vi "Test New File Sink.vi"(11 "Test Case In":refnum<class "File Sink.lvclass">) -> (0 "error out":errorcluster, 3 "Test Case Out":refnum<class "File Sink.lvclass">)   [LabVIEW 2020, in "Testing.lvlib" / "File Sink.lvclass"]
uses:
  File Sink.lvclass
  C:/Program Files (x86)/National Instruments/LabVIEW 2020/vi.lib/Astemes/LUnit/Test Case.lvclass
  Source/Sinks/File Sink/File Sink.lvclass/File Sink.ctl
  <vilib>/Astemes/LUnit/Test Case.lvclass/Test Case.ctl
  4993e8ee-a06a-463a-9684-69129f64d5ce.vi
  <vilib>/Astemes/LUnit/Core/LUnit Test Case/Private/Append Pass Result.vi
  <vilib>/Astemes/LUnit/Core/LUnit Test Case/Private/Append Fail Result.vi
  4993e8ee-a06a-463a-9684-69129f64d5ce.vi/9c5d11cd-9439-4240-a1ee-d9baace9c924.vi
  <vilib>/Astemes/LUnit/Core/LUnit Test Case/Private/Run In UI.vi
  Source/Sinks/File Sink/File Sink.lvclass
  <vilib>/Astemes/LUnit/Test Case.lvclass
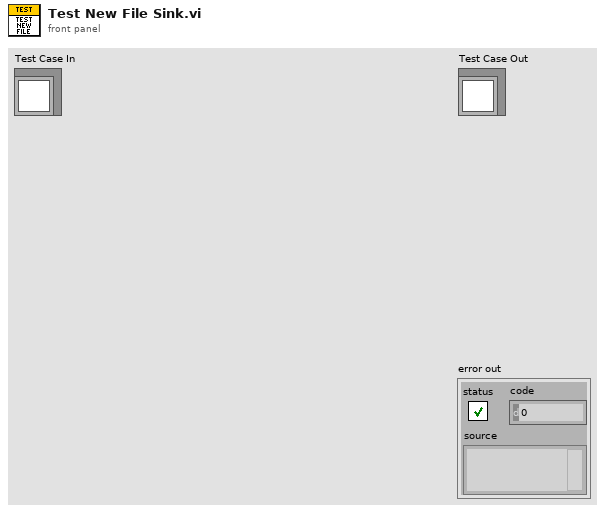
[diagram p1: front panel]
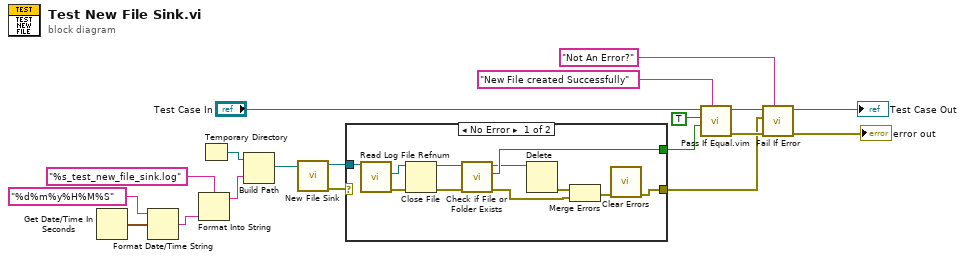
[diagram p0: block diagram]
diagram:
  n1 = Get Date/Time In Seconds() -> (seconds since 1Jan1904=w3:timestamp)
  n2 = Format Date/Time String(time format string (%c)="%d%m%y%H%M%S", seconds (now)=w3) -> (date/time string=w1:string)  [unwired: 1 in]
  n3 = Format Into String(format string="%s_test_new_file_sink.log", w1) -> (resulting string=w4:string)  [unwired: 2 in, 1 out]
  n4 = Temporary Directory() -> (w6:path)
  n5 = Build Path(base path=w6, name or relative path=w4) -> (appended path=w7:path)
  n6 = call "New File Sink.vi"("File Path"=w7) -> ("error out"=w17:errorcluster, "File Sink out"=w18:refnum<class "File Sink.lvclass">)  [unwired: 9 in]
  n7 = case shown="No Error" w17 {
    selector: w17 -> [_ w31]
    tunnel: w18 -> [w30 _]
    tunnel: [w20 w31] -> w9
    tunnel: [w25 _] -> w16
    frame No Error {
      n8 = call "Read Log File Refnum.vi"("File Sink in"=w30) -> ("error out"=w29:errorcluster, "Log File Refnum"=w28:refnum<file>)  [unwired: 8 in, 1 out]
      n9 = Close File(refnum=w28, error in=w29) -> (path=w26:path, error out=w27:errorcluster)
      n10 = call <vilib>:"Check if File or Folder Exists.vi"("error in (no error)"=w27, "path"=w26) -> ("error out"=w22:errorcluster, "file or folder exists?"=w25:bool, "dup path"=w24:path)  [unwired: 7 in]
      n11 = Delete(path (use dialog)=w24) -> (error out=w23:errorcluster)  [unwired: 4 in, 2 out]
      n12 = Merge Errors(w23, w22) -> (w21:errorcluster)
      n13 = call <vilib>:"Clear Errors.vi"("error in (no error)"=w21) -> ("error out"=w20:errorcluster)  [unwired: 5 in, 1 out]
    }
    frame Error {
    }
  }
  n14 = call "Pass If Equal.vim"("Description"="New File created Successfully", "Actual"=w16, "Expected"=TRUE, "LUnit Test Case In"="Test Case In") -> ("error out"=w11:errorcluster, "LUnit Test Case Out"=w13:refnum<class "File Sink.lvclass">)  [unwired: 6 in]
  n15 = call <vilib>:"Fail If Error.vi"("Description"="Not An Error?", "error in (no error)"=w11, "Assert error"=w9, "LUnit Test Case In"=w13) -> ("error out"=→"error out":errorcluster, "LUnit Test Case Out"=→"Test Case Out":refnum<class "File Sink.lvclass">)  [unwired: 6 in]
